vi "Measure Voltage.vi"(8 "error in (no error)":errorcluster, 11 "GEN40-38-LAN in":refnum<class "GEN40-38-LAN.lvclass">) -> (0 "error out":errorcluster, 2 "Voltage":dbl, 3 "GEN40-38-LAN out":refnum<class "GEN40-38-LAN.lvclass">)   [LabVIEW 2018, in "GEN40-38-LAN.lvlib" / "GEN40-38-LAN.lvclass"]
uses:
  GEN40-38-LAN.lvclass
  PPLs/Power Supply/Parent/Power_Supply.lvlibp/Power Supply.lvclass
  C:/Projects/LabVIEW/PPLs/Power Supply/Parent/Power_Supply.lvlibp/Power Supply.lvclass
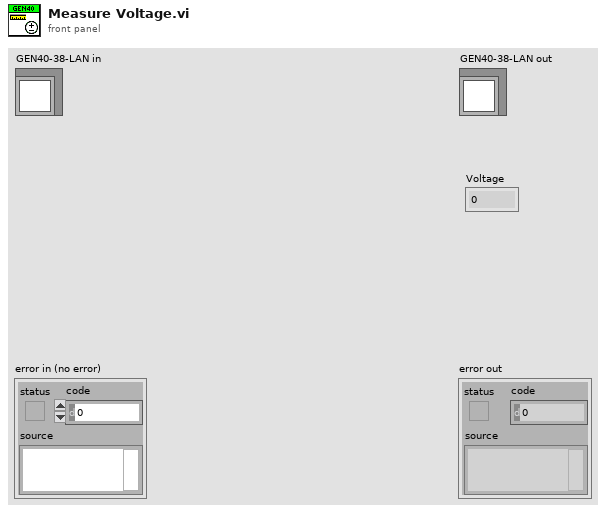
[diagram p1: front panel]
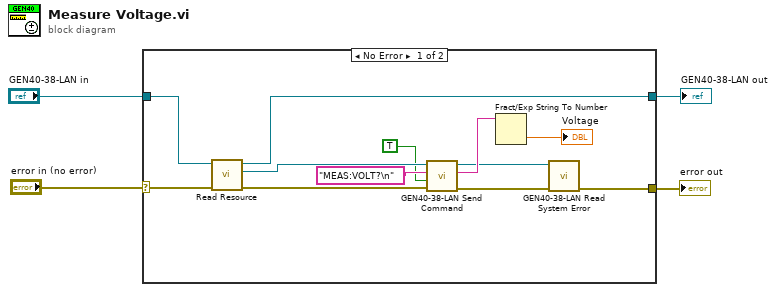
[diagram p0: block diagram]
diagram:
  n1 = case shown="No Error" "error in (no error)" {
    selector: "error in (no error)" -> [w16 w18]
    tunnel: [w5 w18] -> w3
    tunnel: [w13 w17] -> w2
    tunnel: "GEN40-38-LAN in" -> [w15 w17]
    frame No Error {
      n2 = call "Read Resource.vi"("error in"=w16, "Power Supply in"=w15) -> ("error out"=w14:errorcluster, "Resource"=w12:refnum<visa-resource-name>, "Power Supply out"=w13:refnum<class "GEN40-38-LAN.lvclass">)  [unwired: 7 in]
      n3 = call "GEN40-38-LAN Send Command.vi"("error in (no error)"=w14, "Wait for Response?"=TRUE, "Command"="MEAS:VOLT?\n", "VISA resource name"=w12) -> ("error out"=w6:errorcluster, "Response"=w9:string, "VISA resource name out"=w7:refnum<visa-resource-name>)  [unwired: 5 in]
      n4 = Fract/Exp String To Number(string=w9) -> (number=→"Voltage":dbl)  [unwired: 3 in, 1 out]
      n5 = call "GEN40-38-LAN Read System Error.vi"("error in (no error)"=w6, "Resource"=w7) -> ("error out"=w5:errorcluster)  [unwired: 9 in]
    }
    frame Error {
    }
  }
  "error out" <- w3
  "GEN40-38-LAN out" <- w2
